vi "GetType.vi"(8 "error in (no error)":errorcluster, 11 "Configure Trigger Msg":refnum<class "Configure Trigger Msg.lvclass">) -> (0 "error out":errorcluster, 2 "Data Sample":variant, 3 "Configure Trigger Msg":refnum<class "Configure Trigger Msg.lvclass">)   [LabVIEW 2015, in "CS++DMM.lvlib" / "Configure Trigger Msg.lvclass"]
uses:
  Configure Trigger Msg.lvclass
  Configure Trigger Msg.lvclass/Configure Trigger Msg.ctl
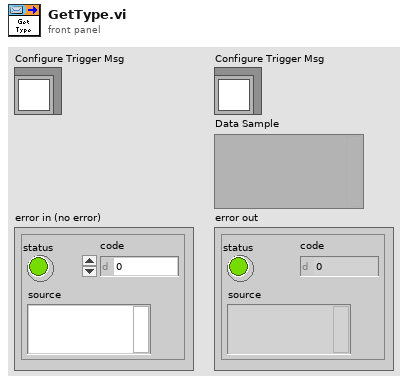
[diagram p1: front panel]
types:
  T1 = cluster{"trigger source (Immediate)":i32, "trigger delay (0.0 s)":dbl}
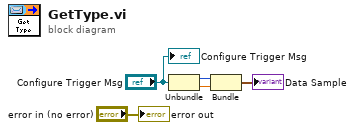
[diagram p0: block diagram]
diagram:
  n1 = Unbundle("Configure Trigger Msg") -> (w2:i32, w1:dbl)
  n2 = Bundle("trigger source (Immediate)"=w2, "trigger delay (0.0 s)"=w1) -> (→"Data Sample":T1)  [unwired: 1 in]
  "error out" <- "error in (no error)"
  "Configure Trigger Msg" <- "Configure Trigger Msg"
